vi "OuputMixer5782.vi"(10 "Phase output":fxp<+,64,64>[](array[numeric])=[0.0, 0.0, 0.0, 0.0], 11 "Signal Input":i16[](array[numeric])=[0, 0]) -> ()   [LabVIEW 2013]
doc: "Mixes input and outputs I and Q on Analog output 0 and 1"
uses:
  <vilib>/rvi/eio/common/nirviEmuTemplateMethod_errors.vi
  <vilib>/eio/EIONode/EIONode.xnode
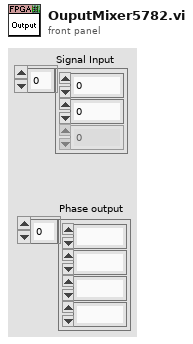
[diagram p1: front panel]
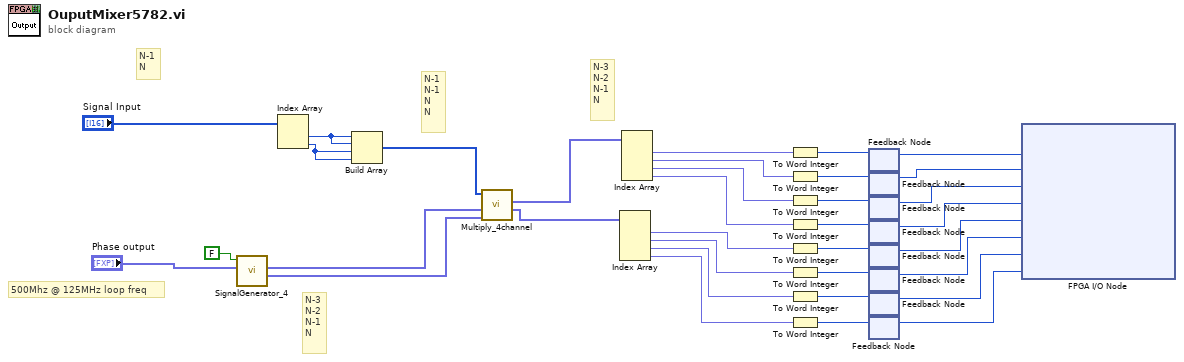
[diagram p0: block diagram]
diagram:
  # "500Mhz @ 125MHz loop freq"
  # "N-3\nN-2\nN-1\nN"
  # "N-3\nN-2\nN-1\nN"
  # "N-1\nN-1\nN\nN"
  # "N-1\nN"
  n1 = call "SignalGenerator_4.vi"("Phase"="Phase output", "reset"=FALSE) -> ("Sine out"=w27:fxp<+/-,16,0>[], "Cosine out"=w28:fxp<+/-,16,0>[])  [unwired: 8 in]
  n2 = Index Array(array="Signal Input") -> (element #1=w31:i16, element #2=w30:i16)  [unwired: 2 in]
  n3 = Build Array(w31, w31, w30, w30) -> (w29:i16[])
  n4 = call "Multiply_4channel.vi"("DDS Sine"=w27, "DDS Cosine"=w28, "Signal Input"=w29) -> ("Q output"=w24:fxp<+/-,16,14>[], "I output"=w26:fxp<+/-,16,14>[])  [unwired: 7 in]
  n5 = Index Array(array=w24) -> (element #1=w20:fxp<+/-,16,14>, element #2=w19:fxp<+/-,16,14>, element #3=w18:fxp<+/-,16,14>, element #4=w17:fxp<+/-,16,14>)  [unwired: 4 in]
  n6 = Index Array(array=w26) -> (element #1=w25:fxp<+/-,16,14>, element #2=w23:fxp<+/-,16,14>, element #3=w22:fxp<+/-,16,14>, element #4=w21:fxp<+/-,16,14>)  [unwired: 4 in]
  n7 = To Word Integer(number=w25) -> (16bit integer=w15:i16)
  n8 = To Word Integer(number=w23) -> (16bit integer=w11:i16)
  n9 = To Word Integer(number=w22) -> (16bit integer=w10:i16)
  n10 = To Word Integer(number=w21) -> (16bit integer=w9:i16)
  n11 = To Word Integer(number=w20) -> (16bit integer=w12:i16)
  n12 = To Word Integer(number=w19) -> (16bit integer=w13:i16)
  n13 = To Word Integer(number=w18) -> (16bit integer=w14:i16)
  n14 = To Word Integer(number=w17) -> (16bit integer=w16:i16)
  n15 = feedback-in #1(w15) -> ()
  n16 = feedback #1() -> (w8:i16)  [unwired: 1 in]
  n17 = feedback #2() -> (w7:i16)  [unwired: 1 in]
  n18 = feedback-in #2(w11) -> ()
  n19 = feedback #3() -> (w6:i16)  [unwired: 1 in]
  n20 = feedback-in #3(w10) -> ()
  n21 = feedback #4() -> (w5:i16)  [unwired: 1 in]
  n22 = feedback-in #4(w9) -> ()
  n23 = feedback #5() -> (w4:i16)  [unwired: 1 in]
  n24 = feedback-in #5(w12) -> ()
  n25 = feedback #6() -> (w3:i16)  [unwired: 1 in]
  n26 = feedback-in #6(w13) -> ()
  n27 = feedback #7() -> (w2:i16)  [unwired: 1 in]
  n28 = feedback-in #7(w14) -> ()
  n29 = feedback #8() -> (w1:i16)  [unwired: 1 in]
  n30 = feedback-in #8(w16) -> ()
  n31 = xnode "FPGA I/O Node"("IO Module\\AO 0 N-3"=w8, "IO Module\\AO 0 N-2"=w7, "IO Module\\AO 0 N-1"=w6, "IO Module\\AO 0 N"=w5, "IO Module\\AO 1 N-3"=w4, "IO Module\\AO 1 N-2"=w3, "IO Module\\AO 1 N-1"=w2, "IO Module\\AO 1 N"=w1) -> ()  [unwired: 8 in, 8 out]
